vi "Switch Cal Standard.vi"(0 "NICal5501 in":refnum<class "Cal Standard.lvclass">, 5 "Standard Type":T1, 7 "Path Name":string, 11 "error in (no error)":errorcluster) -> (4 "NICal5501 out":refnum<class "Cal Standard.lvclass">, 15 "error out":errorcluster)   [LabVIEW 2023, in "NI Cal-5501 Cal Standard.lvlib" / "Cal Standard.lvclass"]
uses:
  Cal Standard.lvclass
  Instruments/Cal Standard/Type Definitions/Standard Type.ctl
  Cal Standard.lvclass/Cal Standard.ctl
  Properties/Read Resource Name.vi
  Properties/Read Product Name.vi
  Common/RFCalAndFixtureCharact.Common.lvlib
  Instruments/RFFixtureCharact.Instruments.lvlib
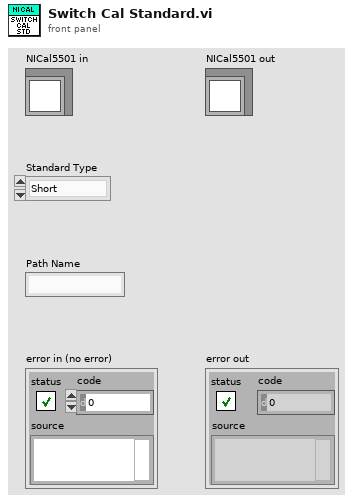
[diagram p1: front panel]
types:
  T1 = typedef "RFFixtureCharact.Instruments.lvlib/Standard Type.ctl" = enum16{"Short", "Open", "Load"}
  T2 = typedef "Standard Control.ctl" = i32
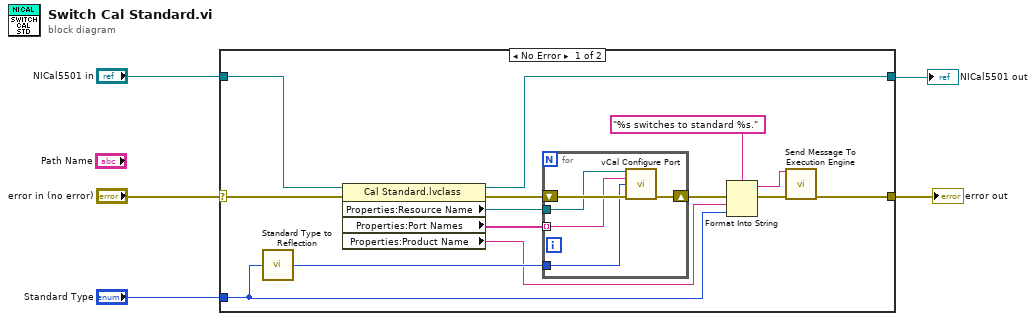
[diagram p0: block diagram]
diagram:
  n1 = case shown="No Error" "error in (no error)" {
    selector: "error in (no error)" -> [w9 w26]
    tunnel: [w15 w26] -> w1
    tunnel: [w18 w25] -> w2
    tunnel: "NICal5501 in" -> [w19 w25]
    tunnel: "Standard Type" -> [w7 _]
    frame No Error {
      n2 = call "Standard Type to Reflection.vi"("Standard Type"=w7) -> ("Standard Type"=w8:T2)
      n3 = property class="Cal Standard.lvclass"(reference=w19, error in=w9) -> (reference out=w18:refnum<class "Cal Standard.lvclass">, error out=w12:errorcluster, "Properties:Resource Name"=w11:refnum<k15>, "Properties:Port Names"=w10:string[], "Properties:Product Name"=w6:string)
      n4 = for {
        tunnel: w8 -> [w22]
        tunnel: w11 -> [w21]
        shift-right: [w24] -> w13
        shift-left: w12 -> [w23]
        tunnel: w10 -> [w20] mode=indexing
        n5 = call <instrlib>:"vCal Configure Port.vi"("instrument handle"=w21, "port name"=w20, "Standard"=w22, "error in"=w23) -> ("error out"=w24:errorcluster)  [unwired: 10 in, 1 out]
      }
      n6 = Format Into String(format string="%s switches to standard %s." ("message"), error in=w13, w6, w7) -> (resulting string=w16:string, error out=w17:errorcluster)  [unwired: 1 in]
      n7 = call "Send Message To Execution Engine.vi"("Message"=w16, "error in (no error)"=w17) -> ("error out"=w15:errorcluster)  [unwired: 13 in]
    }
    frame Error {
    }
  }
  "error out" <- w1
  "NICal5501 out" <- w2
